vi "ff_retag_devices.vi"(8 "error in (no error)":errorcluster) -> (0 "error out":errorcluster, 1 "success rate":bool[](array[boolean]), 2 "address list":string[](array[string]), 3 "deviceID list":string[](array[string]), 4 "new device tags out":string[](array[string]), 5 "total ms":u32, 6 "new device tag numbers out":i32[](array[numeric]))   [LabVIEW 2012]
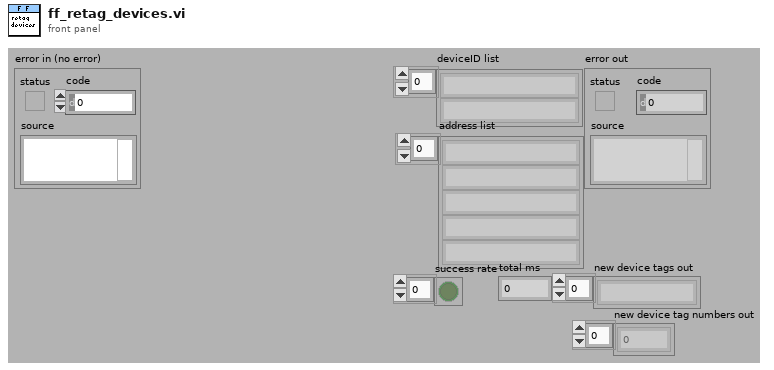
[diagram p1: front panel]
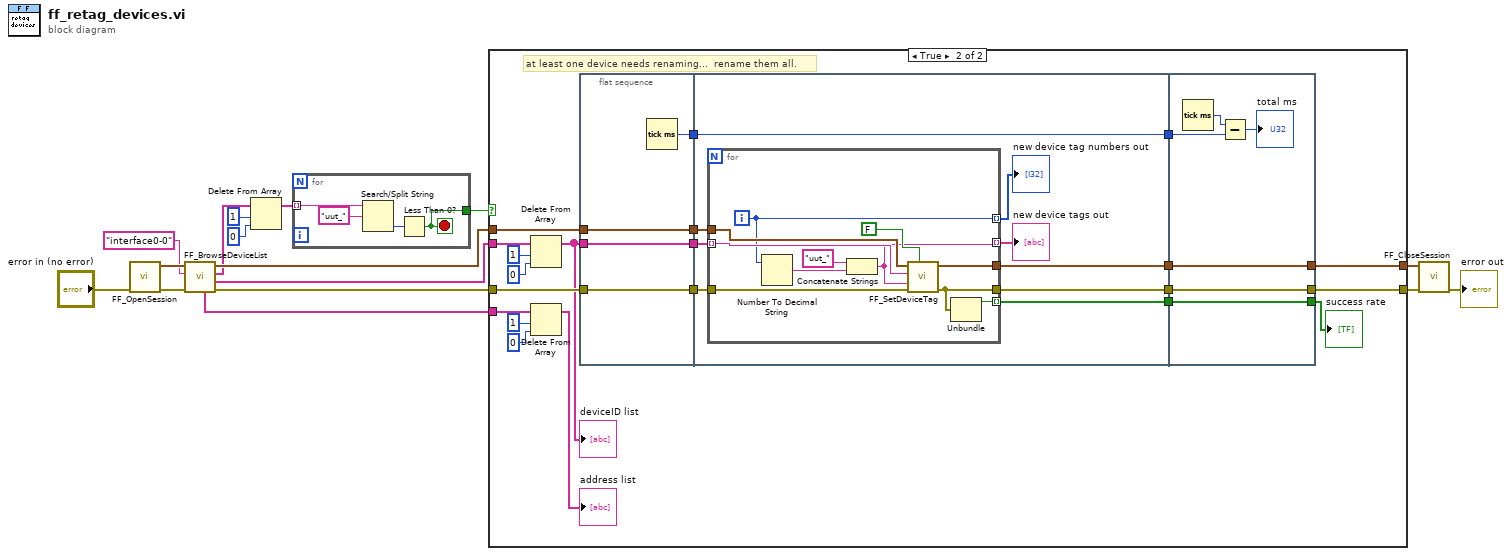
[diagram p0: block diagram]
diagram:
  n1 = call "FF_OpenSession.vi"("error in (no error)"="error in (no error)") -> ("error out"=w15:errorcluster, "refnum out"=w16:cluster{"Handle1":u32, "Handle2":u32})  [unwired: 9 in]
  n2 = call "FF_BrowseDeviceList.vi"("error in (no error)"=w15, "link name"="interface0-0", "refnum in"=w16) -> ("error out"=w12:errorcluster, "deviceID list"=w11:string[], "pdTag list"=w7:string[], "refnum out"=w13:cluster{"Handle1":u32, "Handle2":u32}, "address list"=w10:string[])  [unwired: 4 in]
  n3 = Delete From Array(array=w7, length=1, index=0) -> (array with subset deleted=w5:string[])  [unwired: 1 out]
  n4 = for {
    tunnel: w5 -> [w20] mode=indexing
    tunnel: [w17] -> w1
    stop <- w17 stop-if-true
    n5 = Search/Split String(string=w20, search string/char (-)="uut_") -> (offset of match=w18:i32)  [unwired: 1 in, 2 out]
    n6 = Less Than 0?(x=w18) -> (x < 0?=w17:bool)
  }
  n7 = case shown="True" w1 {
    tunnel: w13 -> [w22 w35]
    tunnel: w12 -> [w21 w34]
    tunnel: w11 -> [_ w30]
    tunnel: w10 -> [_ w26]
    tunnel: [w22 w24] -> w4
    tunnel: [w21 w23] -> w3
    frame False {
    }
    frame True {
      # "at least one device needs renaming...  rename them all."
      n8 = Delete From Array(array=w30, length=1, index=0) -> (array with subset deleted=w29:string[])  [unwired: 1 out]
      "deviceID list" <- w29
      n9 = Delete From Array(array=w26, length=1, index=0) -> (array with subset deleted=→"address list":string[])  [unwired: 1 out]
      n10 = flat-sequence {
        tunnel: w29 -> [w45]
        tunnel: w34 -> [w46]
        tunnel: w35 -> [w47]
        tunnel: [w47] -> w43
        tunnel: [w46] -> w42
        tunnel: [w45] -> w41
        tunnel: [w44] -> w40
        tunnel: w43 -> [w56]
        tunnel: w42 -> [w55]
        tunnel: w41 -> [w54]
        tunnel: [w53] -> w39
        tunnel: [w52] -> w38
        tunnel: [w51] -> w37
        tunnel: w40 -> [w50]
        tunnel: [w50] -> w36
        tunnel: [w71] -> w33
        tunnel: [w72] -> w23
        tunnel: [w73] -> w24
        tunnel: w39 -> [w73]
        tunnel: w38 -> [w72]
        tunnel: w37 -> [w71]
        tunnel: w36 -> [w69]
        frame #0 {
          n11 = Tick Count (ms)() -> (millisecond timer value=w44:u32)
        }
        frame #1 {
          n12 = for {
            tunnel: w56 -> [w67]
            tunnel: w55 -> [w66]
            tunnel: w54 -> [w65] mode=indexing
            tunnel: [w61] -> w53
            tunnel: [w60] -> w52
            tunnel: [w59] -> w51 mode=indexing
            tunnel: [w58] -> w49 mode=indexing
            tunnel: [w57] -> w48 mode=indexing
            i -> [w57]
            n13 = Number To Decimal String(number=w57) -> (decimal integer string=w63:string)  [unwired: 1 in]
            n14 = Concatenate Strings("uut_" ("string"), w63) -> (w58:string)
            n15 = call "FF_SetDeviceTag.vi"("Is pdTag"=FALSE, "error in (no error)"=w66, "new pdTag"=w58, "pdTag/deviceID"=w65, "refnum in"=w67) -> ("error out"=w60:errorcluster, "refnum out"=w61:cluster{"Handle1":u32, "Handle2":u32})  [unwired: 5 in]
            n16 = Unbundle(w60) -> ("status"=w59:bool)  [unwired: 2 out]
          }
          "new device tags out" <- w49
          "new device tag numbers out" <- w48
        }
        frame #2 {
          n17 = Tick Count (ms)() -> (millisecond timer value=w70:u32)
          n18 = Subtract(x=w70, y=w69) -> (x-y=→"total ms":u32)
        }
      }
      "success rate" <- w33
    }
  }
  n19 = call "FF_CloseSession.vi"("error in (no error)"=w3, "refnum in"=w4) -> ("error out"=→"error out":errorcluster)  [unwired: 9 in]
